vi "Test.vi"   [LabVIEW 2016, in "Moving Motor.lvrbt"]
uses:
  Moving Motor.lvrbt
  <vilib>/NXT/Hardware/Plugins/Tetrix DC Motor/TetrixDCMotorAddress.ctl
  <vilib>/NXT/NXTIO Xnodes/NXTIONodeSubVIs/TETRIX IO Move DC Motors.vi
  <vilib>/NXT/NXTIO Xnodes/NXTIONodeSubVIs/TETRIX IO Stop DC Motors.vi
  <vilib>/NXT/Subs/LVHSConnector.ctl
  <vilib>/NXT/NXTIO Xnodes/AddressXNode/NXTIOAddress.xnode
  <vilib>/NXT/NXTIO Xnodes/NXTIOXNode/NXTIO.xnode
  <vilib>/NXT/LegoClasses/BrickReference/BrickReference.lvclass
types:
  T1 = typedef "TetrixDCMotorAddress.ctl" = i32
  T2 = typedef "LVHSConnector.ctl" = refnum<class "BrickReference.lvclass">
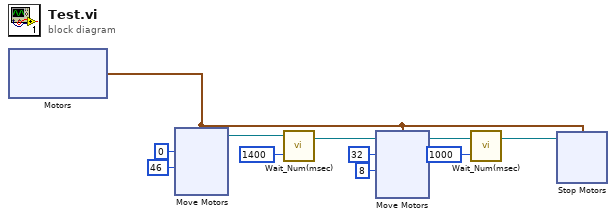
[diagram p0: block diagram]
diagram:
  n1 = xnode "Motors"() -> ("Motor"=w1:cluster{"TetrixDCMotor":T1, "TetrixDCMotor":T1})
  n2 = xnode "Move Motors"("Power/Speed 2"=i8 46, "Power/Speed 1"=i8 0, "Motors"=w1) -> ("NXT/EV3"=w9:T2)  [unwired: 1 in]
  n3 = call <vilib>:"Wait_Num(msec).vi"("Time (100 msec)"=u32 1400, "NXT/EV3"=w9) -> ("NXT/EV3"=w6:T2)  [unwired: 2 in]
  n4 = xnode "Move Motors"("Power/Speed 2"=i8 8, "Power/Speed 1"=i8 32, "Motors"=w1, "NXT/EV3"=w6) -> ("NXT/EV3"=w3:T2)
  n5 = call <vilib>:"Wait_Num(msec).vi"("Time (100 msec)"=u32 1000, "NXT/EV3"=w3) -> ("NXT/EV3"=w2:T2)  [unwired: 2 in]
  n6 = xnode "Stop Motors"("Motors"=w1, "NXT/EV3"=w2) -> ()  [unwired: 1 out]
